vi "change post build step.vi"(7 "CD Execution Mode":T1=enum."Inline Model Interface", 8 "error in (no error)":errorcluster, 10 "User Project":refnum<vi>, 11 "CD Name":string) -> (0 "error out":errorcluster)   [LabVIEW 2014, in "CD model script.lvlib"]
uses:
  CD model script.lvlib
  CD Wizard - Execution Mode.ctl
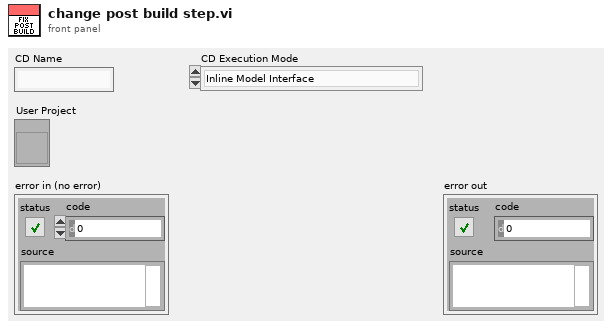
[diagram p1: front panel]
types:
  T1 = typedef "CD model script.lvlib/CD Wizard - Execution Mode.ctl" = enum16{"Asynchronous", "Inline HW Interface", "Inline Model Interface", "Inline Timing and Sync", "Asynchronous Timing and Sync"}
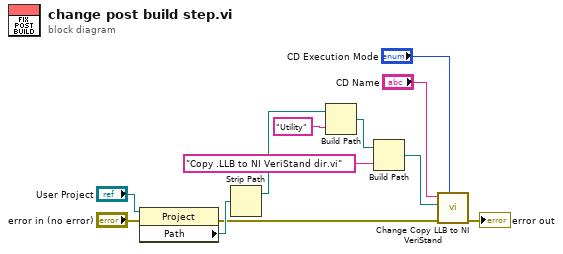
[diagram p0: block diagram]
diagram:
  n1 = property class="Project"(reference="User Project", error in="error in (no error)") -> (error out=w5:errorcluster, "Path"=w7:path)  [unwired: 1 out]
  n2 = Strip Path(path=w7) -> (stripped path=w9:path)  [unwired: 1 out]
  n3 = Build Path(base path=w9, name or relative path="Utility") -> (appended path=w8:path)
  n4 = Build Path(base path=w8, name or relative path="Copy .LLB to NI VeriStand dir.vi") -> (appended path=w12:path)
  n5 = call "Change Copy LLB to NI VeriStand.vi"("CD Execution Mode"="CD Execution Mode", "error in (no error)"=w5, "Copy .LLB to ... path"=w12, "CD Name"="CD Name") -> ("error out"=→"error out":errorcluster)  [unwired: 7 in]
